vi "CANTEST.vi"(0 "DeviceType":T1=3 items=["PCI-CAN200"=7, "USB-CAN"=2, "USB-CAN200"=3], 1 "kCanBaud":u8(ring)=12 items=["250k bps"=10, "10k bps"=2, "5k bps"=1, "50k bps"=5, "40k bps"=4, "20k bps"=3, "80k bps"=6, "100k bps"=7, "125k bps"=8, "200k bps"=9, "400k bps"=11, "500k bps"=12, "666k bps"=13, "800k bps"=14, "1000k bps"=15], 5 "CANChannel":u32, 7 "DevInd":u32, 9 "ID(Hex 高位有效)":string="00000182", 11 "错误输入":errorcluster caption="错误输入（无错误）", 12 "Data Input(Hex)":string="000007d100000000") -> (4 "帧数据":string, 8 "Result":bool, 10 "Time":u32, 15 "错误输出":errorcluster)   [LabVIEW 2013]
uses:
  DevType.ctl
  InitConfig.ctl
  Global.vi
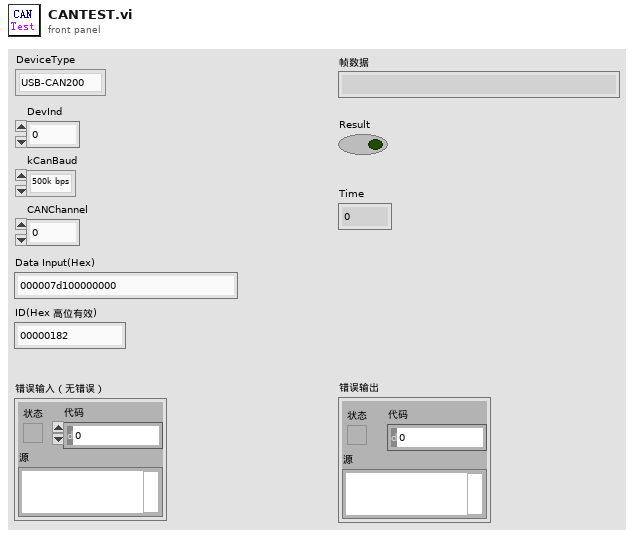
[diagram p1: front panel]
types:
  T1 = typedef "DevType.ctl" = u16
  T2 = typedef "InitConfig.ctl" = cluster{"AccCode":u32, "AccMask":u32, "Reserved":u32, "Filter":u8, "kCanBaud":u8, "Timing0":u8, "Timing1":u8, "Mode":u8, "CanRx_IER":u8}
  T3 = cluster{"ID":u8, u8, u8, u8, "TimeStamp":u32, "TimeFlag":u8, "SendType":u8, "RemoteFlag":u8, "ExternFlag":u8, "DataLen":u8, "Byte0":u8, "Byte1":u8, "Byte2":u8, "Byte3":u8, "Byte4":u8, "Byte5":u8, "Byte6":u8, "Byte7":u8, "Channel":u8, u8, u8}
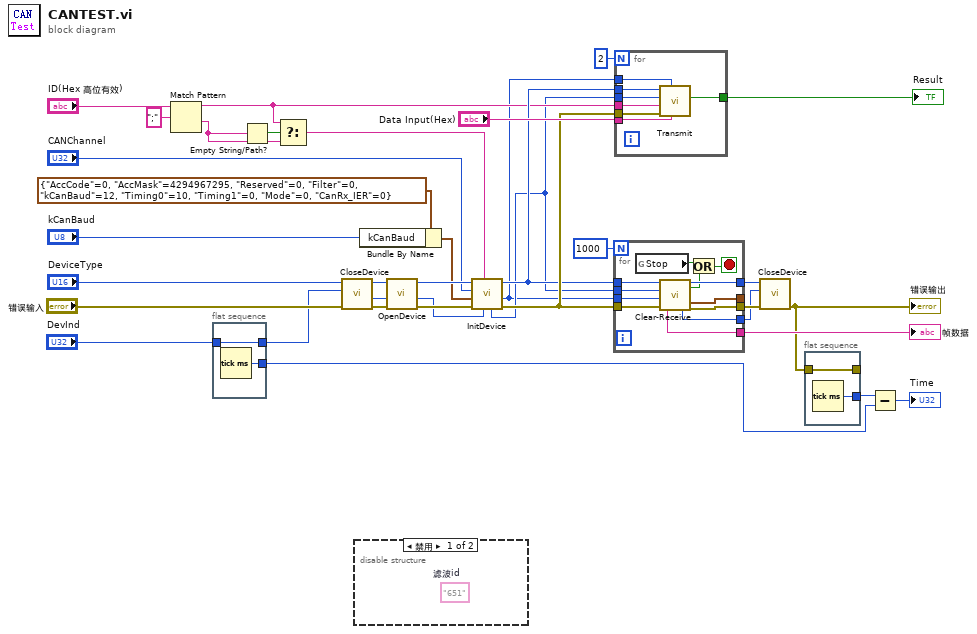
[diagram p0: block diagram]
diagram:
  n1 = Match Pattern(string="ID(Hex 高位有效)", regular expression=";" ("正则表达式")) -> (before substring=w18:string, after substring=w17:string)  [unwired: 1 in, 2 out]
  n2 = flat-sequence {
    tunnel: "DevInd" -> [w38]
    tunnel: [w38] -> w5
    tunnel: [w37] -> w2
    frame #0 {
      n3 = Tick Count (ms)() -> (millisecond timer value=w37:u32)
    }
  }
  n4 = Empty String/Path?(string/path=w17) -> (empty?=w19:bool)
  n5 = Select(t=w18, s=w19, f=w17) -> (s? t:f=w16:string)
  n6 = call "CloseDevice.vi"("错误输入（无错误）"="错误输入", "DevInd"=w5, "DeviceType"="DeviceType") -> ("错误输出"=w30:errorcluster, "DeviceInd"=w15:u32, "DeviceTypeOut"=w35:T1)  [unwired: 5 in, 1 out]
  n7 = disable-structure shown="禁用" {
    frame Disabled {
      (unwired) "651"  # 滤波id
    }
    frame Enabled {
    }
  }
  n8 = Bundle By Name(cluster=T2 {"AccCode"=0, "AccMask"=4294967295, "Reserved"=0, "Filter"=0, "kCanBaud"=12, "Timing0"=10, "Timing1"=0, "Mode"=0, "CanRx_IER"=0} ("InitConfig"), "kCanBaud"="kCanBaud") -> (w7:T2)
  n9 = call "OpenDevice.vi"("错误输入（无错误）"=w30, "DevInd"=w15, "DeviceType"=w35) -> ("错误输出"=w31:errorcluster, "DevIndex"=w14:u32, "DeviceTypeOut"=w34:T1)  [unwired: 5 in, 1 out]
  n10 = call "InitDevice.vi"("DevInd"=w14, "ID(Hex 高位有效)"=w16, "错误输入"=w31, "InitConfig"=w7, "CanChannel"="CANChannel", "DeviceType"=w34) -> ("错误输出"=w26:errorcluster, "DevIndex"=w11:u32, "DeviceTypeOut"=w23:T1, "CanIndex"=w12:u32)  [unwired: 1 in, 1 out]
  n11 = for {
    N: 1000 -> [_]
    tunnel: w12 -> [w44]
    tunnel: w26 -> [w50]
    tunnel: [w49] -> _
    tunnel: [w48] -> w27
    tunnel: [w47] -> w25
    tunnel: w23 -> [w46]
    tunnel: [w45] -> w24
    tunnel: w11 -> [w43]
    tunnel: [w42] -> w10
    stop <- w39 stop-if-true
    n12 = global read "Global.vi" "Stop"() -> (w40:bool)
    n13 = call "Clear-Receive.vi"("DeviceType"=w46, "CANChannel"=w44, "DevInd"=w43, "错误输入"=w50) -> ("data"=w47:string, "DeviceInd"=w42:u32, "DeviceTypeOut"=w45:T1, "Result"=w41:bool, "VCI_CAN_OBJ_R"=w49:T3, "错误输出"=w48:errorcluster)  [unwired: 7 in, 3 out]
    n14 = Or(x=w40, y=w41) -> (x .or. y?=w39:bool)
  }
  "帧数据" <- w25
  n15 = for {
    N: 2 -> [_]
    tunnel: [w57] -> w33
    tunnel: w18 -> [w56]
    tunnel: "Data Input(Hex)" -> [w55]
    tunnel: w12 -> [w54]
    tunnel: w26 -> [w53]
    tunnel: w23 -> [w52]
    tunnel: w11 -> [w51]
    n16 = call "Transmit.vi"("Data Input(Hex)"=w55, "DevInd"=w51, "错误输入"=w53, "ID(Hex 高位有效)"=w56, "CANChannel"=w54, "DeviceType"=w52) -> ("Result"=w57:bool)  [unwired: 1 in, 4 out]
  }
  "Result" <- w33
  n17 = call "CloseDevice.vi"("错误输入（无错误）"=w27, "DevInd"=w10, "DeviceType"=w24) -> ("错误输出"=w4:errorcluster)  [unwired: 5 in, 3 out]
  "错误输出" <- w4
  n18 = flat-sequence {
    tunnel: w4 -> [w59]
    tunnel: [w59] -> _
    tunnel: [w58] -> w3
    frame #0 {
      n19 = Tick Count (ms)() -> (millisecond timer value=w58:u32)
    }
  }
  n20 = Subtract(x=w3, y=w2) -> (x-y=→"Time":u32)
